vi "CheckBuildFolder.vi"(1 "appended path":path) -> ()   [LabVIEW 2014]
doc: "Checks permissions to determine whether or not data folders can be created"
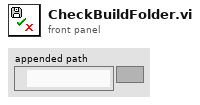
[diagram p1: front panel]
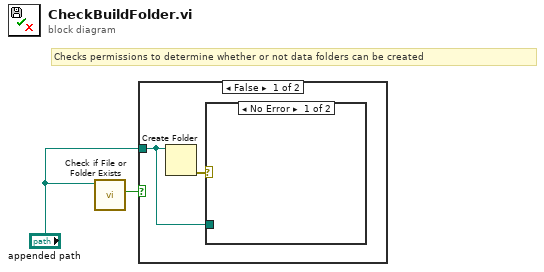
[diagram p0: block diagram]
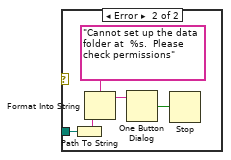
[diagram p2: hidden frame]
diagram:
  # "Checks permissions to determine whether or not data folders can be created"
  n1 = call <vilib>:"Check if File or Folder Exists.vi"("path"="appended path") -> ("file or folder exists?"=w1:bool)  [unwired: 8 in, 2 out]
  n2 = case shown="False" w1 {
    tunnel: "appended path" -> [w3 _]
    frame False {
      n3 = Create Folder(path (use dialog)=w3) -> (error out=w4:errorcluster)  [unwired: 2 in, 2 out]
      n4 = case shown="No Error" w4 {
        tunnel: w3 -> [_ w6]
        frame No Error {
        }
        frame Error {
          n5 = Path To String(path=w6) -> (string=w5:string)
          n6 = Format Into String(format string="Cannot set up the data folder at  %s.  Please check permissions" ("name or relative path"), w5) -> (resulting string=w7:string)  [unwired: 2 in, 1 out]
          n7 = One Button Dialog(message=w7) -> (true=w9:bool)  [unwired: 1 in]
          n8 = Stop(stop? (T)=w9) -> ()
        }
      }
    }
    frame True {
    }
  }
